vi "命令输出.vi"(8 "error in (no error)":errorcluster caption="错误输入（无错误）", 11 "TimingControl 输入":refnum<class "TimingControl.lvclass">) -> (0 "error out":errorcluster caption="错误输出", 2 "数据":cluster{"启动":bool, "控制命令":T1, "测量参数":T2}={"启动"=FALSE, "控制命令"=enum."加标回收（启动采配水）", "测量参数"={"氨氮"=TRUE, "总磷"=TRUE, "总氮"=TRUE, "CODMn"=TRUE, "CODCr"=FALSE, "氟化物"=FALSE, "挥发酚"=FALSE}}, 3 "TimingControl 输出":refnum<class "TimingControl.lvclass">)   [LabVIEW 2016, in "ZKTimingControl.lvlib" / "TimingControl.lvclass"]
uses:
  TimingControl.lvclass
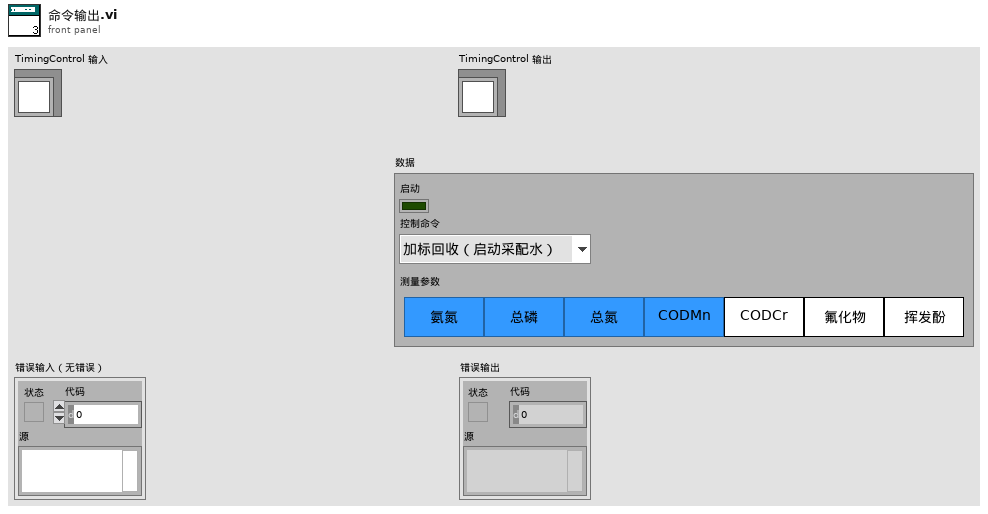
[diagram p1: front panel]
types:
  T1 = typedef "ZKTimingControl.lvlib/TimingControl.lvclass/国标控制命令.ctl" = enum16{"加标回收（启动采配水）", "加标回收（不启动采配水）", "水样测试（启动采配水）", "水样测试（不启动采配水）", "平行样测试（启动采配水）", "平行样测试（不启动采配水）", "集成干预测试"}
  T2 = typedef "ZKTimingControl.lvlib/TimingControl.lvclass/测量参数.ctl" = cluster{"氨氮":bool, "总磷":bool, "总氮":bool, "CODMn":bool, "CODCr":bool, "氟化物":bool, "挥发酚":bool}
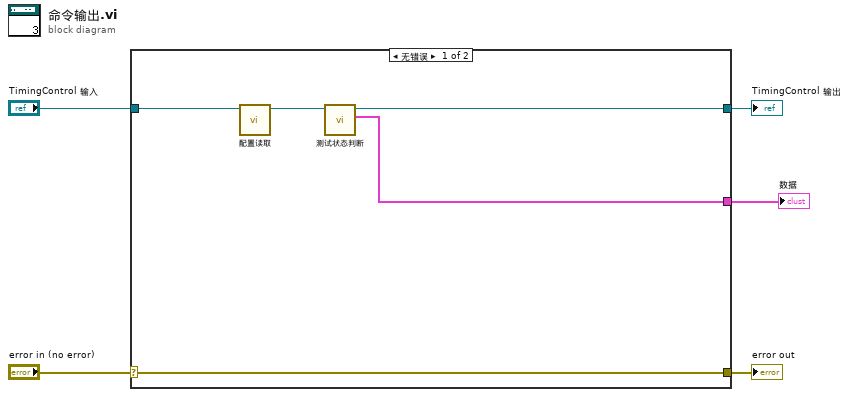
[diagram p0: block diagram]
diagram:
  n1 = case shown="无错误" "error in (no error)" {
    selector: "error in (no error)" -> [w10 w12]
    tunnel: [w10 w12] -> w4
    tunnel: [w7 w11] -> w2
    tunnel: "TimingControl 输入" -> [w6 w11]
    tunnel: [w9 _] -> w1
    frame No Error {
      n2 = call "配置读取.vi"("TimingControl 输入"=w6) -> ("TimingControl 输出"=w8:refnum<class "TimingControl.lvclass">)  [unwired: 9 in, 1 out]
      n3 = call "测试状态判断.vi"("TimingControl 输入"=w8) -> ("数据"=w9:cluster{"启动":bool, "控制命令":T1, "测量参数":T2}, "TimingControl 输出"=w7:refnum<class "TimingControl.lvclass">)  [unwired: 9 in]
    }
    frame Error {
    }
  }
  "error out" <- w4
  "TimingControl 输出" <- w2
  "数据" <- w1
